vi "Parser.vi"(8 "error in (no error)":errorcluster, 9 "flatten cluster? (F)":bool, 11 "variant":variant) -> (0 "error out":errorcluster, 3 "parameters":T1[](array[typedef]))   [LabVIEW 2011]
uses:
  <vilib>/addons/database/Auxilliary.llb/DB Tools Parameter Info.ctl
  <vilib>/addons/database/Auxilliary.llb/DB Tools DataTypes.ctl
  <vilib>/addons/database/Auxilliary.llb/DB Tools Parameter Dir.ctl
  <vilib>/Utility/VariantDataType/VariantType.lvlib
  <vilib>/addons/database/NI_Database_API.lvlib
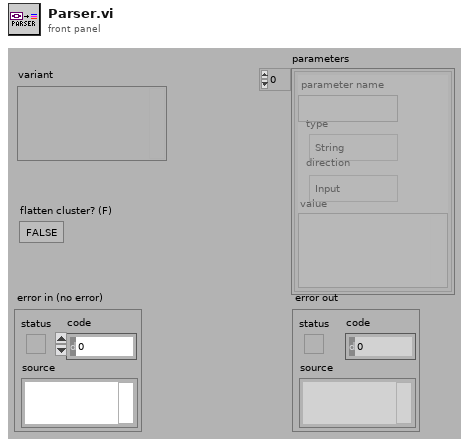
[diagram p1: front panel]
types:
  T1 = typedef "NI_Database_API.lvlib/DB Tools Parameter Info.ctl" = cluster{"parameter name":string, "type":T2, "direction":T3, "value":variant}
  T2 = typedef "NI_Database_API.lvlib/DB Tools DataTypes.ctl" = enum16{"String", "Long (I32)", "Single (SGL)", "Double (DBL)", "Date/Time", "Binary"}
  T3 = typedef "NI_Database_API.lvlib/DB Tools Parameter Dir.ctl" = enum32{"Input", "Output", "Input/Output", "Return Value"}
  T4 = typedef "VariantType.lvlib/Type.ctl" = enum8{"Invalid Type", "Void", "I8", "I16", "I32", "I64", "U8", "U16", "U32", "U64", "Single Float", "Double Float", "Extended Float", "Single Complex", "Double Complex", "Extended Complex", "Enum U8", "Enum U16", "Enum U32", "Enum U64", "Single Float With Unit", "Double Float With Unit", "Extended Float With Unit", "Single Complex with Unit", "Double Complex with Unit", "Extended Complex with Unit", "Boolean", "String", "Path", "Picture", "Tag", "Array", "Cluster", "Variant", "LV Variant", "Waveform", "Timestamp", "Digital Waveform", "Digital Data", "ExpressData", "Refnum", "External Data", "VI", "Poly VI", "LabVIEW Class Instance", "Fixed Point"}
  T5 = cluster{"parameter name":string, "type":T2, "direction":T3, "value":variant}
  T6 = cluster{"parameter name":string, "type":T2, "direction":T3, "value":variant}[]
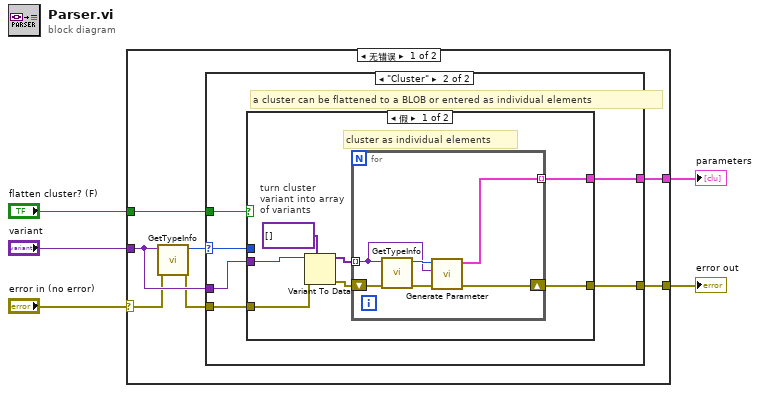
[diagram p0: block diagram]
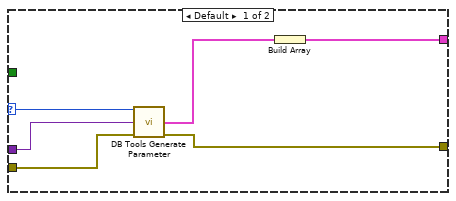
[diagram p2: hidden frame]
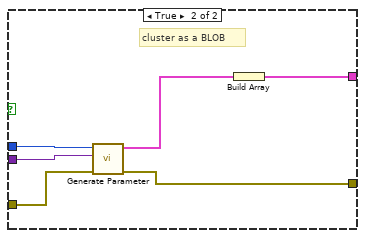
[diagram p3: hidden frame]
diagram:
  n1 = case shown="无错误" "error in (no error)" {
    selector: "error in (no error)" -> [w7 w44]
    tunnel: [w12 w44] -> w2
    tunnel: "variant" -> [w10 _]
    tunnel: [w9 _] -> w4
    tunnel: "flatten cluster? (F)" -> [w8 _]
    frame No Error {
      n2 = call <vilib>:"GetTypeInfo.vi"("error in (no error)"=w7, "Variant"=w10) -> ("error out"=w6:errorcluster, "Type Enum"=w11:T4)  [unwired: 5 in, 3 out]
      n3 = case shown="\"Cluster\"" w11 {
        selector: w11 -> [w18 w19]
        tunnel: [w15 w21] -> w12
        tunnel: [w13 w23] -> w9
        tunnel: w6 -> [w16 w22]
        tunnel: w10 -> [w17 w20]
        tunnel: w8 -> [_ w24]
        frame Default {
          n4 = call <vilib>:"DB Tools Generate Parameter.vi"("Type Enum"=w18, "Variant data"=w17, "error in (no error)"=w16) -> ("parameter information"=w14:T1, "error out"=w15:errorcluster)  [unwired: 11 in]
          n5 = Build Array(w14) -> (w13:T1[])
        }
        frame "Cluster" {
          # "a cluster can be flattened to a BLOB or entered as individual elements"
          n6 = case shown="假" w24 {
            tunnel: [w25 w40] -> w23
            tunnel: w22 -> [w28 w39]
            tunnel: [w26 w38] -> w21
            tunnel: w20 -> [w31 w42]
            tunnel: w19 -> [_ w43]
            frame False {
              # "cluster as individual elements"
              # "turn cluster variant into array of variants"
              n7 = Variant To Data(error in=w28, type=variant[] [], Variant=w31) -> (data=w29:variant[], error out=w27:errorcluster)
              n8 = for {
                tunnel: w29 -> [w34] mode=indexing
                shift-right: [w33] -> w26
                shift-left: w27 -> [w35]
                tunnel: [w32] -> w25 mode=indexing
                n9 = call <vilib>:"GetTypeInfo.vi"("error in (no error)"=w35, "Variant"=w34) -> ("error out"=w36:errorcluster, "Type Enum"=w37:T4)  [unwired: 5 in, 3 out]
                n10 = call "Generate Parameter.vi"("error in (no error)"=w36, "Variant data"=w34, "Type Enum"=w37) -> ("error out"=w33:errorcluster, "parameter information"=w32:T5)  [unwired: 7 in]
              }
            }
            frame True {
              # "cluster as a BLOB"
              n11 = call "Generate Parameter.vi"("error in (no error)"=w39, "Variant data"=w42, "Type Enum"=w43) -> ("error out"=w38:errorcluster, "parameter information"=w41:T5)  [unwired: 7 in]
              n12 = Build Array(w41) -> (w40:T6)
            }
          }
        }
      }
    }
    frame Error {
    }
  }
  "error out" <- w2
  "parameters" <- w4
